vi "Create.vi"(6 "Image Type":T1, 7 "Border":i32=3, 8 "error in":errorcluster, 11 "Image Name":string) -> (0 "error out":errorcluster, 3 "Image Reference Out":T2)   [LabVIEW 2020, in "OpenLvVision_Image.lvlib" / "Management.lvlib"]
doc: "Creates a new image reference with the specified, unique name. This allocates memory to hold image data and returns a reference for subsequent image processing operations."
uses:
  Management.lvlib
  TypeDef/Image.ctl
  TypeDef/ImageType.ctl
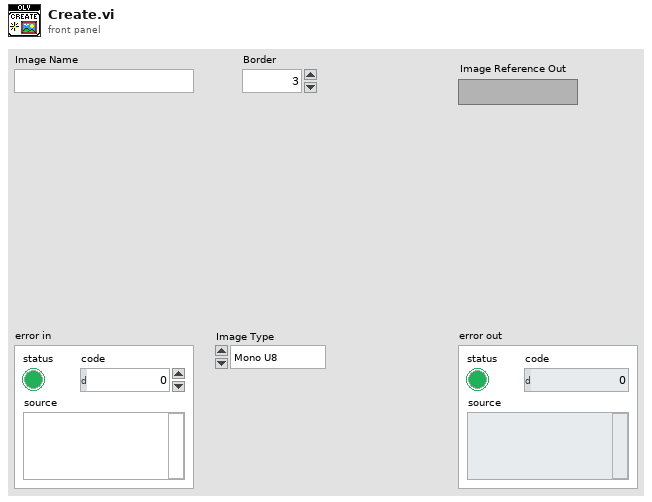
[diagram p1: front panel]
types:
  T1 = typedef "OpenLvVision_Image.lvlib/Management.lvlib/ImageType.ctl" = enum16{"Mono U8", "Mono U16", "Mono I16", "Mono SGL", "Color U32", "Color U64", "Complex CSG"}
  T2 = typedef "OpenLvVision_Image.lvlib/Management.lvlib/Image.ctl" = refnum<image>
  T3 = typedef "Image Type" = u32
  T4 = typedef "IMAQ Image.ctl" = refnum<image>
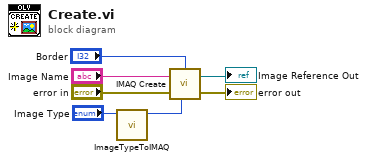
[diagram p0: block diagram]
diagram:
  n1 = call "ImageTypeToIMAQ.vi"("OLV Image Type"="Image Type") -> ("IMAQ Image Type"=w3:T3)  [unwired: 10 in]
  n2 = call "IMAQ Create"("Border Size"="Border", "Image Name"="Image Name", "Image Type"=w3, "error in (no error)"="error in") -> ("New Image"=→"Image Reference Out":T4, "error out"=→"error out":errorcluster)  [unwired: 1 in]
